vi "UI Event Handler.vi"() -> ()   [LabVIEW 2012]
uses:
  <vilib>/Utility/miscctls.llb/LVPoint32TypeDef.ctl
panel:
  out "current time":timestamp
  in  "Time Check":bool
  out "Coords":T1
  out "Iteration":i32
  in  "Stop":bool
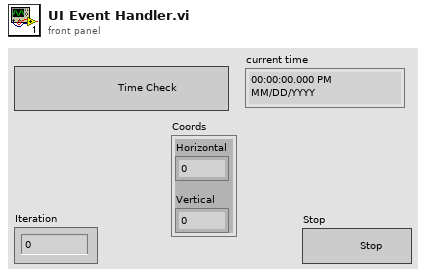
[diagram p1: front panel]
types:
  T1 = typedef "LVPoint32TypeDef.ctl" = cluster{"Horizontal":i32, "Vertical":i32}
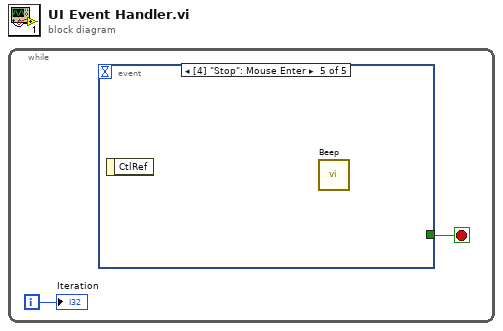
[diagram p0: block diagram]
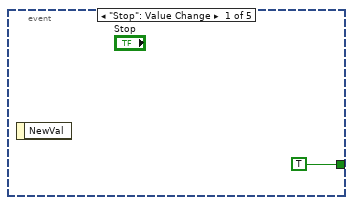
[diagram p2: hidden frame]
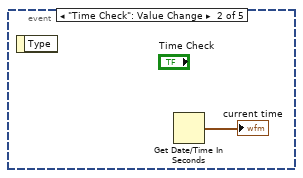
[diagram p3: hidden frame]
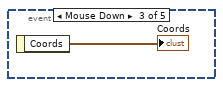
[diagram p4: hidden frame]
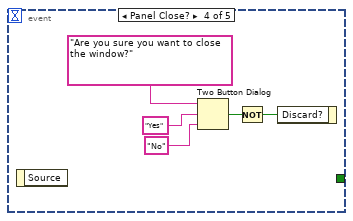
[diagram p5: hidden frame]
diagram:
  n1 = while {
    i -> [w2]
    stop <- w1 stop-if-true
    n2 = event shown="[4] \"Stop\": Mouse Enter" {
      selector: _ -> [_ _ _ _ _]
      dyn-events: _ -> [_ _ _ _ _]
      timeout: _ -> [_ _ _ _ _]
      tunnel: [TRUE _ _ _ _] -> w1
      event "Stop": Value Change {
        n3 = event-data() -> ()  [unwired: 1 in, 1 out]
      }
      event "Time Check": Value Change {
        n4 = event-data() -> ()  [unwired: 1 in, 1 out]
        n5 = Get Date/Time In Seconds() -> (seconds since 1Jan1904=→"current time":timestamp)
      }
      event Mouse Down {
        n6 = event-data() -> ("Coords"=→"Coords":T1)  [unwired: 1 in]
      }
      event Panel Close? {
        n7 = event-data() -> ()  [unwired: 1 in, 1 out]
        n8 = Two Button Dialog(message="Are you sure you want to close the window?", 1:"No" ("T button name (\"OK\")"), 2:"Yes" ("F button name (\"Cancel\")")) -> (T button?=w10:bool)
        n9 = Not(x=w10) -> (.not. x?=w6:bool)
        n10 = event-data("Discard?"=w6) -> ()  [unwired: 1 in, 1 out]
      }
      event "Stop": Mouse Enter {
        n11 = event-data() -> ()  [unwired: 1 in, 1 out]
        n12 = call <vilib>:"Beep.vi"() -> ()  [unwired: 12 in]
      }
    }
    "Iteration" <- w2
  }
